vi "test Open Client No Listener.vi"(8 "error in (no error)":errorcluster, 11 "TestCase in":refnum<class "test Secure Socket.lvclass">) -> (0 "error out":errorcluster, 3 "TestCase out":refnum<class "test Secure Socket.lvclass">)   [LabVIEW 2013, in "test Secure Socket.lvclass"]
uses:
  test Secure Socket.lvclass
  SSL_Lib/SSL-Context/SSL Verify Mode.ctl
  SSL_Lib/SSL-Context/SSL Options.ctl
  SSL_Lib/SSL-Lib/Library Paths.ctl
  SSL Client Context/SSL Client Context.lvclass/SSL Client Context.ctl
  SSL Client Context/SSL Client Context.lvclass
  SSL Client Socket/SSL Client Socket.lvclass
  SSL Client Context/Write Verification Options.vi
  SSL Client Context/Write Verification CA Bundle Path.vi
  SSL Client Context/Write SSL Options.vi
  SSL Client Context/Write Cipher List.vi
  <vilib>/addons/_JKI Toolkits/VI Tester/TestCase.llb/TestCase.lvclass
  SSL_Lib/SSL-Context/SSL-Context.lvclass
  SSL_Lib/SSL-Lib/SSL-Lib.lvclass
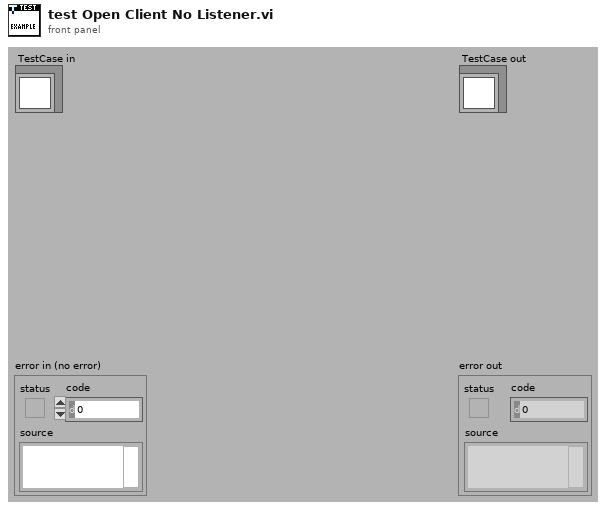
[diagram p1: front panel]
types:
  T1 = typedef "SSL_Lib.lvlib/SSL-Lib.lvclass/Library Paths.ctl" = cluster{"SSL Library Path":path, "Crypto Library Path":path}
  T2 = typedef "SSL_Lib.lvlib/SSL-Context.lvclass/SSL Options.ctl" = i32
  T3 = typedef "SSL_Lib.lvlib/SSL-Context.lvclass/SSL Verify Mode.ctl" = i32
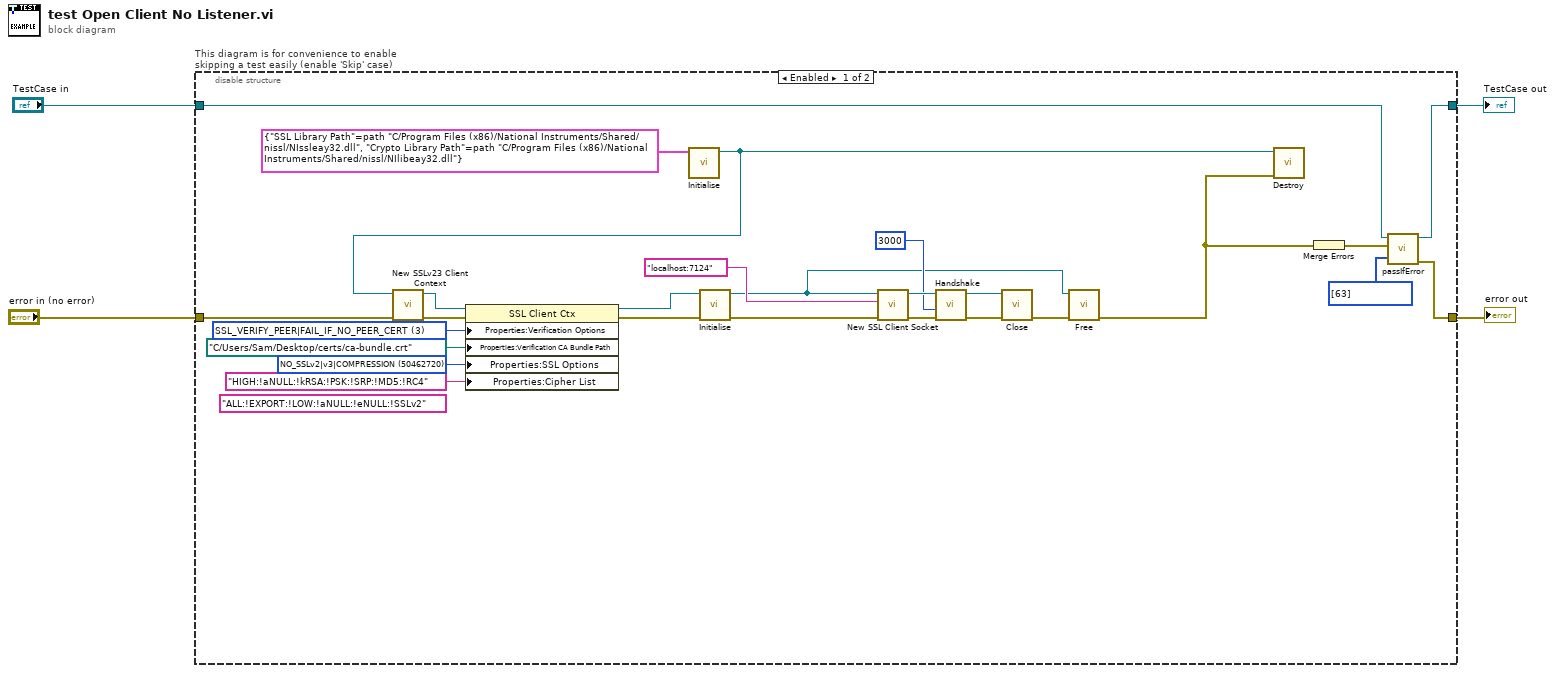
[diagram p0: block diagram]
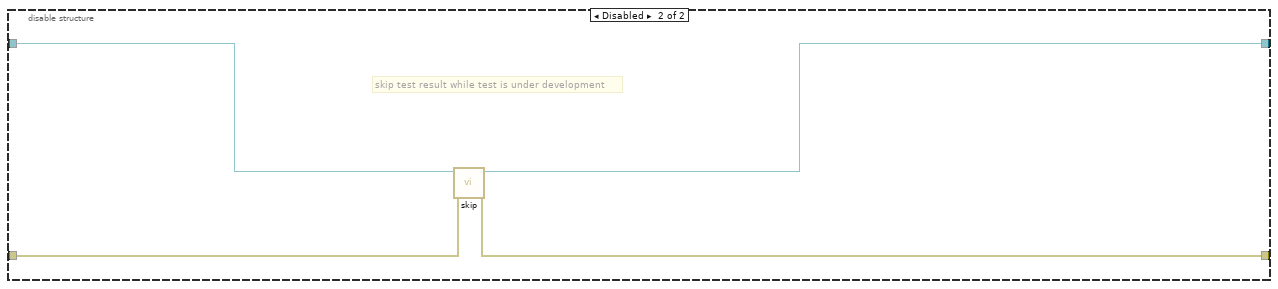
[diagram p2: hidden frame]
diagram:
  n1 = disable-structure "This diagram is for convenience to enable skipping a test easily (enable 'Skip' case)" shown="Enabled" {
    disable-tunnel: "TestCase in" -> [w28 w34]
    disable-tunnel: [w30 w32] -> w1
    disable-tunnel: [w29 w33] -> w3
    disable-tunnel: "error in (no error)" -> [w20 w31]
    frame Enabled {
      (unwired) "ALL:!EXPORT:!LOW:!aNULL:!eNULL:!SSLv2" ("Cipher List")
      w21 = T2 50462720 items=["None"=0, "NO_SSLv2|v3|COMPRESSION"=50462720, "SSL_OP_NO_COMPRESSION"=131072, "SSL_OP_NO_SSLv2"=16777216, "SSL_OP_NO_SSLv3"=33554432, "SSL_OP_NO_TLSv1"=67108864, "SSL_OP_NO_TLSv1_2"=134217728, "SSL_OP_NO_TLSv1_1"=268435456] ("SSL Options")
      w23 = T3 3 items=["SSL_VERIFY_PEER|FAIL_IF_NO_PEER_CERT"=3, "SSL_VERIFY_NONE"=0, "SSL_VERIFY_PEER"=1, "SSL_VERIFY_FAIL_IF_NO_PEER_CERT"=2, "SSL_VERIFY_CLIENT_ONCE"=4] ("Verification Options")
      n2 = call "Initialise.vi"("Library Paths"=T1 {"SSL Library Path"=path "C:/Program Files (x86)/National Instruments/Shared/nissl/NIssleay32.dll", "Crypto Library Path"=path "C:/Program Files (x86)/National Instruments/Shared/nissl/NIlibeay32.dll"}) -> ("SSL-Lib out"=w5:refnum<class "SSL-Lib.lvclass">)  [unwired: 9 in, 1 out]
      n3 = call "New SSLv23 Client Context.vi"("error in (no error)"=w20, "SSL-Lib"=w5) -> ("error out"=w27:errorcluster, "SSL Client Context out"=w25:refnum<class "SSL Client Context.lvclass">)  [unwired: 8 in]
      n4 = property class="SSL Client Ctx"(reference=w25, error in=w27, "Properties:Verification Options"=w23, "Properties:Verification CA Bundle Path"=path "C:/Users/Sam/Desktop/certs/ca-bundle.crt" ("Path to CA bundle"), "Properties:SSL Options"=w21, "Properties:Cipher List"="HIGH:!aNULL:!kRSA:!PSK:!SRP:!MD5:!RC4" ("Cipher List")) -> (reference out=w24:refnum<class "SSL Client Context.lvclass">, error out=w26:errorcluster)
      n5 = call-dynamic "Initialise.vi"("error in (no error)"=w26, "OpenSSL Client Context in"=w24) -> ("error out"=w16:errorcluster, "OpenSSL Client Context out"=w10:refnum<class "SSL Client Context.lvclass">)  [unwired: 8 in]
      n6 = call "New SSL Client Socket.vi"("error in (no error)"=w16, "Hostname / URL"="localhost:7124", "SSL Client Ctx"=w10) -> ("error out"=w17:errorcluster, "SSL Client Skt out"=w18:refnum<class "SSL Client Socket.lvclass">)  [unwired: 7 in]
      n7 = call-dynamic "Handshake.vi"("error in (no error)"=w17, "Timeout (5000ms)"=u32 3000, "OpenSSL in"=w18) -> ("error out"=w13:errorcluster, "OpenSSL out"=w12:refnum<class "SSL Client Socket.lvclass">)  [unwired: 7 in]
      n8 = call-dynamic "Close.vi"("error in (no error)"=w13, "OpenSSL Socket in"=w12) -> ("error out"=w11:errorcluster)  [unwired: 9 in]
      n9 = call-dynamic "Free.vi"("error in (no error)"=w11, "OpenSSL Context in"=w10) -> ("error out"=w6:errorcluster)  [unwired: 9 in]
      n10 = call "Destroy.vi"("error in (no error)"=w6, "SSL-Lib in"=w5) -> ()  [unwired: 9 in, 1 out]
      n11 = Merge Errors(w6) -> (w8:errorcluster)
      n12 = call-dynamic "passIfError.vi"("passing error codes (default = any error code)"=i32[] [63], "error"=w8, "TestCase in"=w28) -> ("error out"=w29:errorcluster, "TestCase out"=w30:refnum<class "test Secure Socket.lvclass">)  [unwired: 7 in]
    }
    frame Disabled {
      # "skip test result while test is under development"
      n13 = call <vilib>:"skip.vi"("error in (no error)"=w31, "TestCase in"=w34) -> ("error out"=w33:errorcluster, "TestCase out"=w32:refnum<class "test Secure Socket.lvclass">)  [unwired: 8 in]
    }
  }
  "error out" <- w3
  "TestCase out" <- w1
